vi "RogersLog.vi"(0 "Text to add":string, 1 "ROS":T3, 2 "Log":T2, 3 "LogPath in":path, 4 "Task":T1(ring)=enum."Add Task") -> (5 "HTML":string, 6 "LogPath out":path)   [LabVIEW 2012]
uses:
  <userlib>/ROSforLV/ROS/Code/SubVIs/_ROSControl.ctl
  <userlib>/ROSforLV/ROS/Code/SubVIs/_ROSDirection.ctl
  <userlib>/ROSforLV/ROS/Code/Console/Servers/ServerSubs/ROSLog.ctl
panel:
  out "Counter":i32
  out "call chain":string[](array[string])
  # "First line is the Menu name - rest is a reamble."
  # "Changed log typedef and then all the registrations"
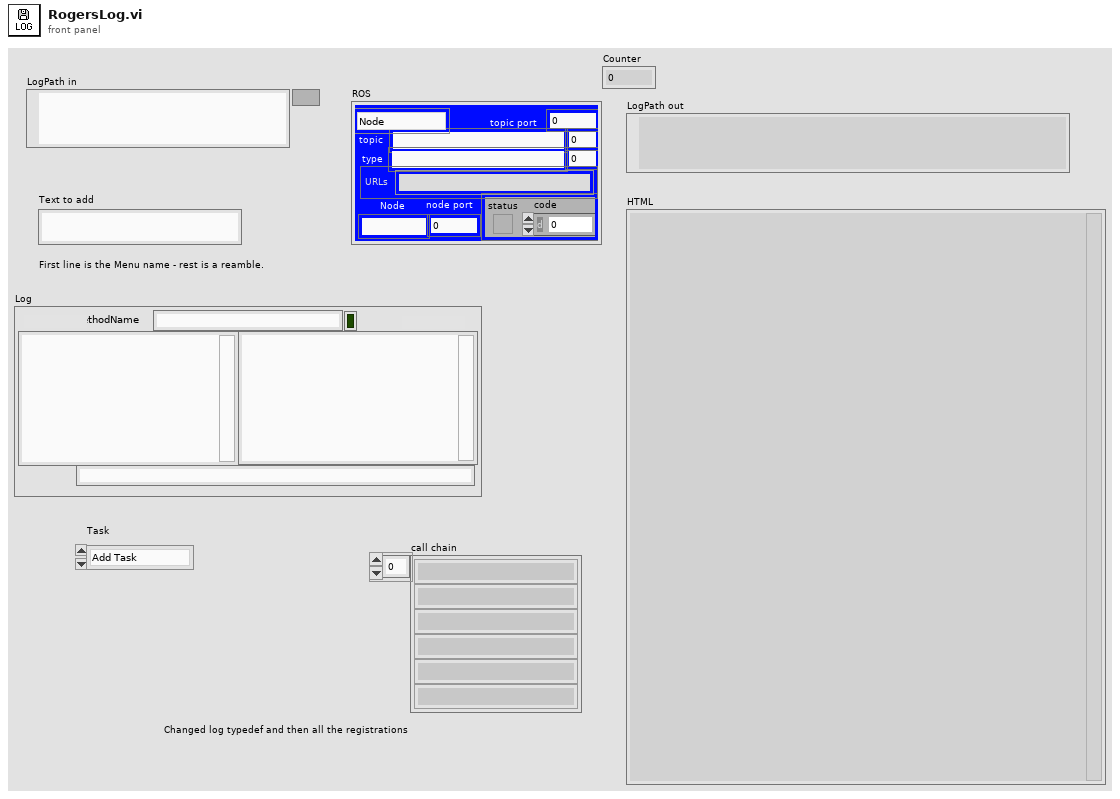
[diagram p1: front panel]
types:
  T1 = enum16{"Reset Log", "Add Client", "Remove Client", "Add Task"}
  T2 = typedef "ROSLog.ctl" = cluster{"Sent":string, "Reply":string, "MethodName":string, "success":bool, "Dir1":string, "Dir2":string, "Time Stamp":string, "error":errorcluster, "Preamble":string}
  T3 = typedef "_ROSControl.ctl" = cluster{"topic port":u16, "Node":string, "topic":string, "type":string, "node port":u32, "error ":errorcluster, "Direction":T4, "APIs":string[], "Update (ms)":u16, "write queue":u16}
  T4 = typedef "_ROSDirection.ctl" = enum16{"Node", "Publisher", "Subscriber", "Service Client"}
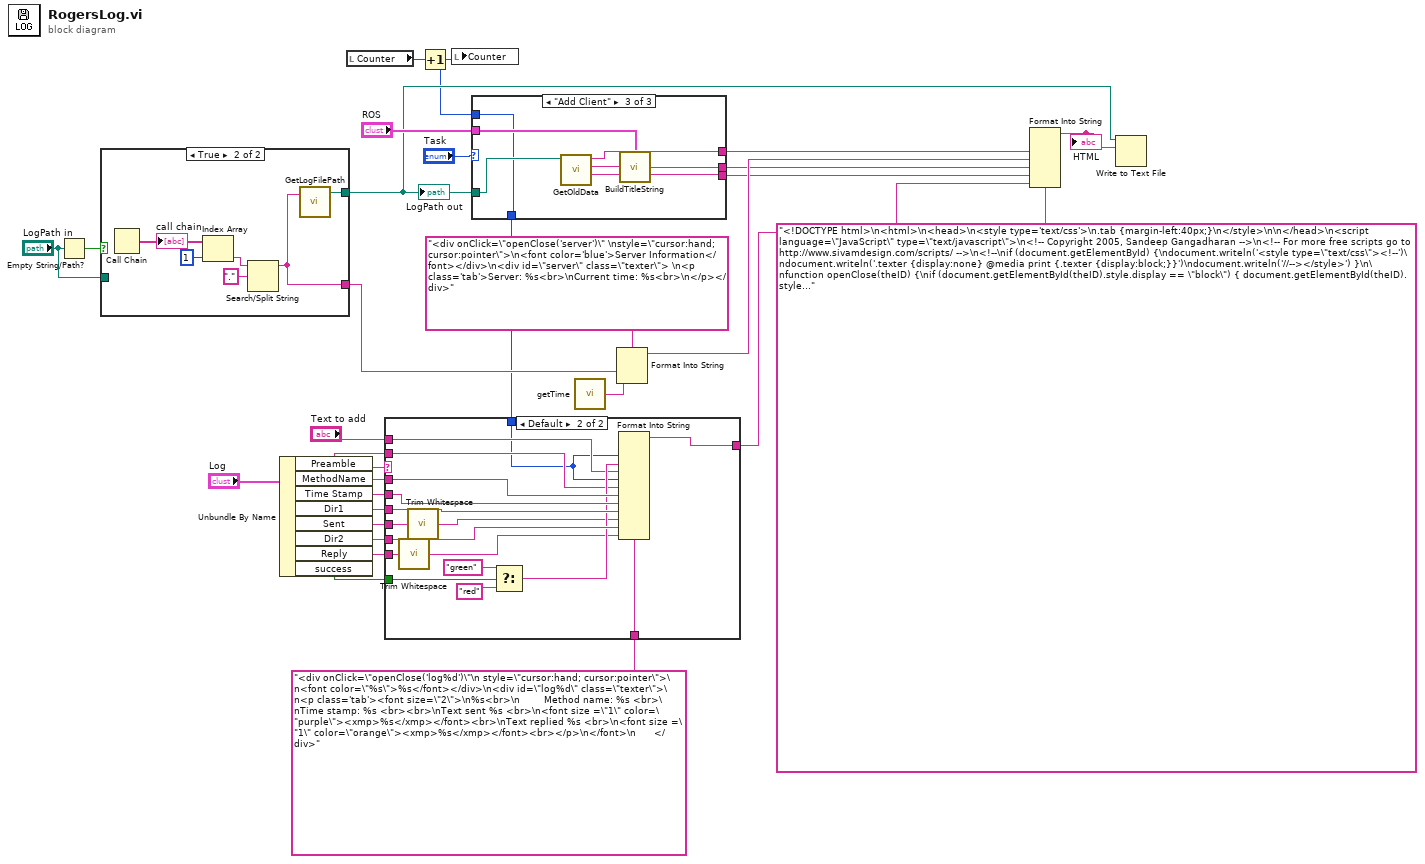
[diagram p0: block diagram]
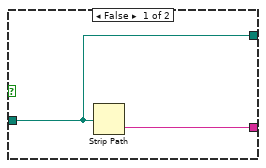
[diagram p2: hidden frame]
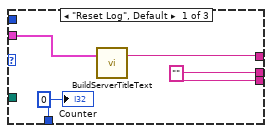
[diagram p3: hidden frame]
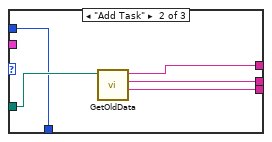
[diagram p4: hidden frame]
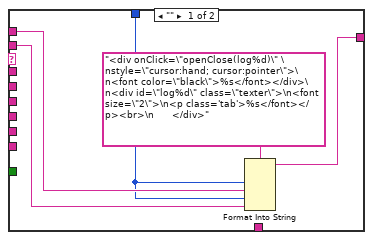
[diagram p5: hidden frame]
diagram:
  n1 = Empty String/Path?(string/path="LogPath in") -> (empty?=w9:bool)
  n2 = case shown="True" w9 {
    tunnel: [w31 w33] -> w8
    tunnel: "LogPath in" -> [w30 _]
    tunnel: [w30 w32] -> w6
    frame False {
      n3 = Strip Path(path=w30) -> (name=w31:string)  [unwired: 1 out]
    }
    frame True {
      n4 = Call Chain() -> (call chain=w34:string[])
      "call chain" <- w34
      n5 = Index Array(array=w34, index=1) -> (element=w37:string)
      n6 = Search/Split String(string=w37, search string/char (-)=".") -> (substring before match=w33:string)  [unwired: 1 in, 2 out]
      n7 = call <userlib>:"GetLogFilePath.vi"("Server name"=w33) -> ("LogPath"=w32:path)  [unwired: 1 in, 1 out]
    }
  }
  "LogPath out" <- w6
  n8 = Unbundle By Name("Log") -> ("Preamble"=w5:string, "MethodName"=w15:string, "Time Stamp"=w26:string, "Dir1"=w25:string, "Sent"=w24:string, "Dir2"=w23:string, "Reply"=w22:string, "success"=w16:bool)
  n9 = local read "Counter"() -> (w2:i32)
  n10 = Increment(x=w2) -> (x+1=w1:i32)
  n11 = local write "Counter"(w1) -> ()
  n12 = case shown="\"Add Client\"" "Task" {
    tunnel: [w41 w44 w51] -> w17
    tunnel: [w39 w46 w53] -> w14
    tunnel: [w41 w43 w49] -> w11
    tunnel: w6 -> [_ w45 w52]
    tunnel: "ROS" -> [w40 _ w48]
    tunnel: [w38 w42 w47] -> w3
    tunnel: w1 -> [_ w42 w47]
    frame "Reset Log", Default {
      w38 = 0
      w41 = "" ("tagged text")
      n13 = call <userlib>:"BuildServerTitleText.vi"("ROS"=w40) -> ("colored text"=w39:string)  [unwired: 1 in, 1 out]
      "Counter" <- w38
    }
    frame "Add Task" {
      n14 = call <userlib>:"GetOldData.vi"("LogPath"=w45) -> ("log"=w44:string, "clients"=w43:string, "server"=w46:string)  [unwired: 8 in]
    }
    frame "Add Client" {
      n15 = call <userlib>:"GetOldData.vi"("LogPath"=w52) -> ("log"=w51:string, "clients"=w50:string, "server"=w53:string)  [unwired: 8 in]
      n16 = call <userlib>:"BuildTitleString.vi"("tagged text"=w50, "ROS"=w48) -> ("String"=w49:string)
    }
  }
  n17 = case shown="Default" w15 {
    tunnel: "<div onClick=\"openClose('log%d')\"\n style=\"cursor:hand; cursor:pointer\">\n<font color=\"%s\">%s</font></div>\n<div id=\"log%d\" class=\"texter\">\n<p class='tab'><font size=\"2\">\n%s<br>\n        Method name: %s <br>\nTime stamp: %s <br><br>\nText sent %s <br>\n<font size =\"1\" color=\"purple\"><xmp>%s</xmp></font><br>\nText replied %s <br>\n<font size =\"1\" color=\"orange\"><xmp>%s</xmp></font><br></p>\n</font>\n      </div>" ("regular expression") -> [_ w75]
    tunnel: w15 -> [_ w74]
    tunnel: w26 -> [_ w73]
    tunnel: w25 -> [_ w72]
    tunnel: w24 -> [_ w71]
    tunnel: w23 -> [_ w70]
    tunnel: w22 -> [_ w69]
    tunnel: [w58 w68] -> w20
    tunnel: w16 -> [_ w65]
    tunnel: "Text to add" -> [w56 w63]
    tunnel: w5 -> [w55 w60]
    tunnel: w3 -> [w54 w59]
    frame "" {
      n18 = Format Into String(format string="<div onClick=\"openClose(log%d)\" \nstyle=\"cursor:hand; cursor:pointer\">\n<font color=\"black\">%s</font></div>\n<div id=\"log%d\" class=\"texter\">\n<font size=\"2\">\n<p class='tab'>%s</font></p><br>\n      </div>" ("regular expression"), w54, w56, w54, w55) -> (resulting string=w58:string)  [unwired: 2 in, 1 out]
    }
    frame Default {
      n19 = call <vilib>:"Trim Whitespace.vi"("string"=w69) -> ("trimmed string"=w61:string)  [unwired: 1 in]
      n20 = call <vilib>:"Trim Whitespace.vi"("string"=w71) -> ("trimmed string"=w62:string)  [unwired: 1 in]
      n21 = Select(t="green" ("format string"), s=w65, f="red" ("format string")) -> (s? t:f=w64:string)
      n22 = Format Into String(format string=w75, w59, w64, w63, w59, w60, w74, w73, w72, w62, w70, w61) -> (resulting string=w68:string)  [unwired: 2 in, 1 out]
    }
  }
  n23 = call <userlib>:"getTime.vi"() -> ("Current Time"=w13:string)  [unwired: 1 in]
  n24 = Format Into String(format string="<div onClick=\"openClose('server')\" \nstyle=\"cursor:hand; cursor:pointer\">\n<font color='blue'>Server Information</font></div>\n<div id=\"server\" class=\"texter\"> \n<p class='tab'>Server: %s<br>\nCurrent time: %s<br>\n</p></div>" ("regular expression"), w8, w13) -> (resulting string=w18:string)  [unwired: 2 in, 1 out]
  n25 = Format Into String(format string="<!DOCTYPE html>\n<html>\n<head>\n<style type='text/css'>\n.tab {margin-left:40px;}\n</style>\n\n</head>\n<script language=\"JavaScript\" type=\"text/javascript\">\n<!-- Copyright 2005, Sandeep Gangadharan -->\n<!-- For more free scripts go to http://www.sivamdesign.com/scripts/ -->\n<!--\nif (document.getElementById) {\ndocument.writeln('<style type=\"text/css\"><!--')\ndocument.writeln('.texter {display:none} @media print {.texter {display:block;}}')\ndocument.writeln('//--></style>') }\n\nfunction openClose(theID) {\nif (document.getElementById(theID).style.display == \"block\") { document.getElementById(theID).style.display = \"none\" }\nelse { document.getElementById(theID).style.display = \"block\" } }\n// -->\n</script>\n\n<body>\n<a href='index.html'>Return to console</a>\n<!----- start server ----->\n%s \n<!----- end server ----->\n \n%s\n<!----- start clients ----->\n%s\n<!----- end clients ----->\n<hr>\n<!----- start log ----->      \n%s\n%s\n<!----- end log ----->\n\n\n</body>\n</html>" ("regular expression"), w14, w18, w11, w17, w20) -> (resulting string=w19:string)  [unwired: 2 in, 1 out]
  "HTML" <- w19
  n26 = Write to Text File(file (use dialog)=w6, text=w19) -> ()  [unwired: 2 in, 3 out]
